vi "JTAG Special Test.vi"(8 "error in (no error)":errorcluster, 11 "Ring":u16(ring)=200 items=["Ram Continous Read"=200, "Ram Continous Write"=201, "MSP430 RAM Test"=202, "MSP430 RESETB Test"=203, "Saturn Start BC"=204, "<Reserved 1>"=205, "<Reserved 2>"=206, "<Reserved 3>"=207, "<Reserved 4>"=208, "<Reserved 5>"=209]) -> (0 "error out":errorcluster)   [LabVIEW 2010]
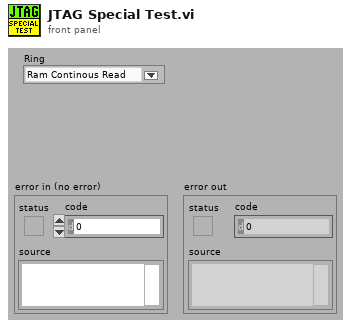
[diagram p1: front panel]
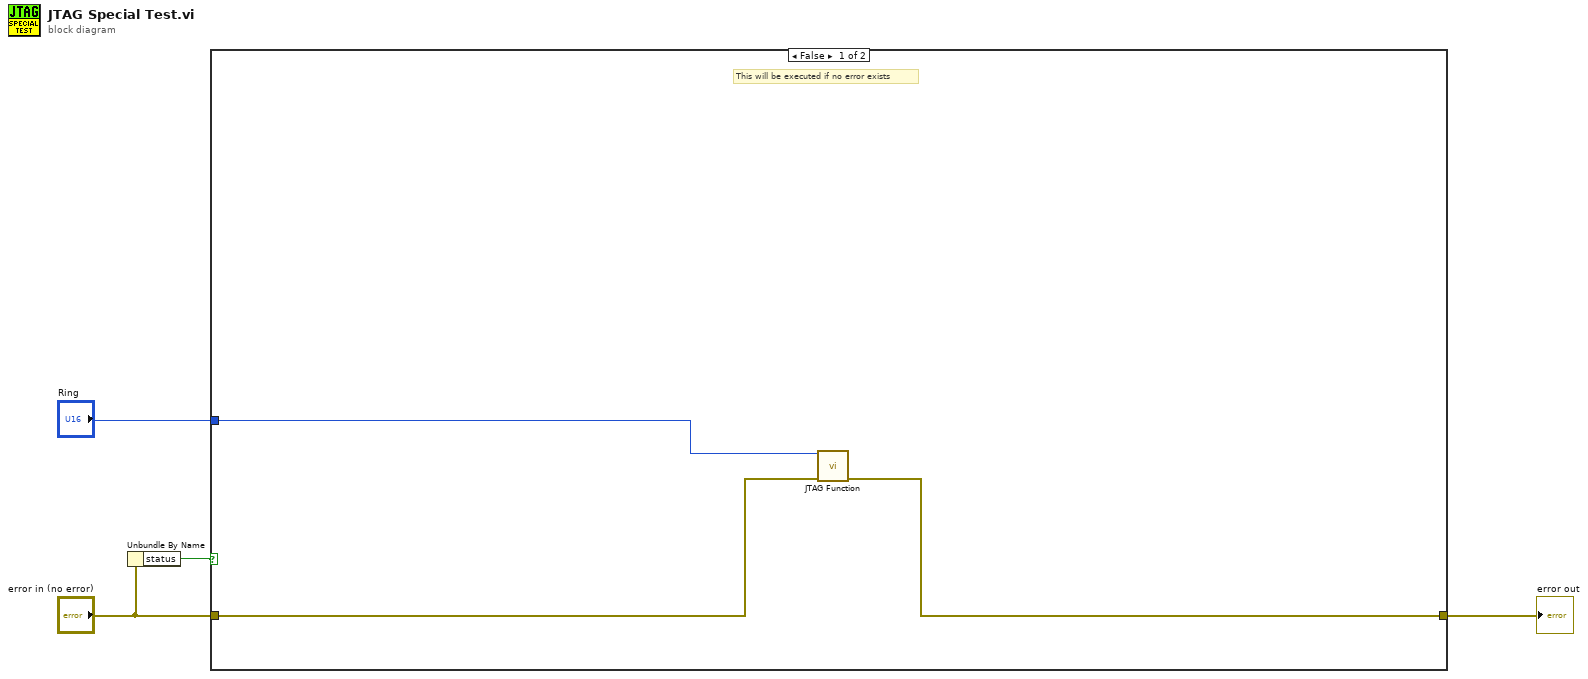
[diagram p0: block diagram]
diagram:
  n1 = Unbundle By Name("error in (no error)") -> ("status"=w3:bool)
  n2 = case shown="False" w3 {
    tunnel: [w6 w8] -> w4
    tunnel: "error in (no error)" -> [w7 w8]
    tunnel: "Ring" -> [w5 _]
    frame False {
      # "This will be executed if no error exists"
      n3 = call "JTAG Function.vi"("Enum"=w5, "error in (no error)"=w7) -> ("error out"=w6:errorcluster)  [unwired: 11 in, 2 out]
    }
    frame True {
      # "Error exists, skip all functions"
    }
  }
  "error out" <- w4
